vi "Add Field to Image.vi"(9 "Terminal Info":T1, 10 "location":i16=1, 11 "picture":picture) -> (3 "new picture":picture)   [LabVIEW 2015, in "LVJSON.lvlib" / "Set Object Parameters.xnode"]
uses:
  Set Object Parameters.xnode
  offsets.vi
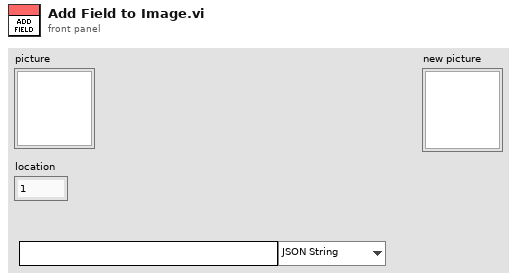
[diagram p1: front panel]
types:
  T1 = cluster{"Parameter Name":string, "JSON Type":enum16{"JSON String", "JSON Numeric", "JSON Boolean", "JSON", "JSON Object", "JSON Array", "String Value", "Numeric Value", "Boolean Value"}}
  T2 = enum16{"User-specified Font", "Application Font", "System Font", "Dialog Font"}
  T3 = cluster{"Font Name:":string, "Size":i16, "Strikeout?":bool, "Italic?":bool, "Underline?":bool, "Outline?":bool, "Shadow?":bool, "Bold?":bool}
  T4 = cluster{"left":i16, "top":i16, "right":i16, "bottom":i16}
  T5 = enum16{"JSON String", "JSON Numeric", "JSON Boolean", "JSON", "JSON Object", "JSON Array", "String Value", "Numeric Value", "Boolean Value"}
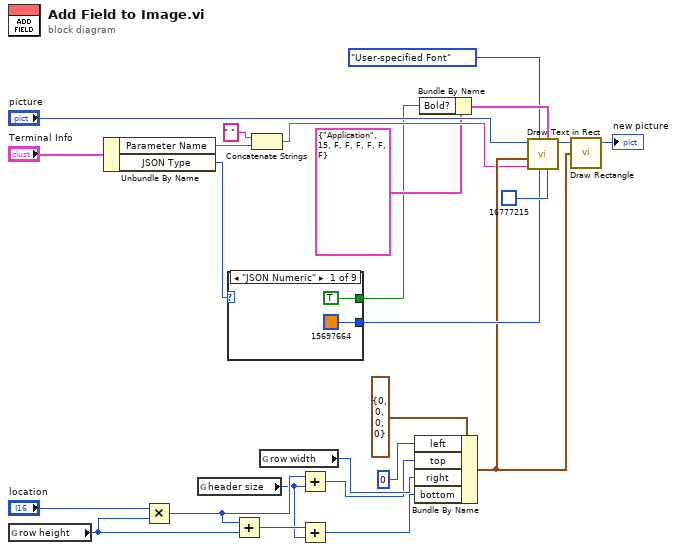
[diagram p0: block diagram]
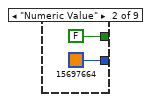
[diagram p2: hidden frame]
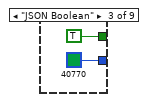
[diagram p3: hidden frame]
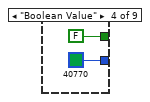
[diagram p4: hidden frame]
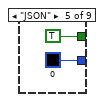
[diagram p5: hidden frame]
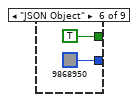
[diagram p6: hidden frame]
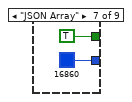
[diagram p7: hidden frame]
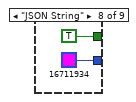
[diagram p8: hidden frame]
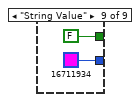
[diagram p9: hidden frame]
diagram:
  n1 = global read "offsets.vi" "row height"() -> (w22:i16)
  n2 = Unbundle By Name("Terminal Info") -> ("Parameter Name"=w7:string, "JSON Type"=w12:T5)
  n3 = Multiply(x="location", y=w22) -> (x*y=w17:i16)
  n4 = global read "offsets.vi" "header size"() -> (w16:i16)
  n5 = case shown="\"JSON Numeric\"" w12 {
    tunnel: [u32 15697664 ("text color(black)") u32 15697664 ("text color(black)") u32 40770 ("text color(black)") u32 40770 ("text color(black)") u32 0 ("text color(black)") u32 9868950 ("text color(black)") u32 16860 ("text color(black)") u32 16711934 ("text color(black)") u32 16711934 ("text color(black)")] -> w10
    tunnel: [TRUE FALSE TRUE FALSE TRUE TRUE TRUE TRUE FALSE] -> w3
    frame "JSON Numeric" {
    }
    frame "Numeric Value" {
    }
    frame "JSON Boolean" {
    }
    frame "Boolean Value" {
    }
    frame "JSON" {
    }
    frame "JSON Object" {
    }
    frame "JSON Array" {
    }
    frame "JSON String" {
    }
    frame "String Value" {
    }
  }
  n6 = Add(x=w17, y=w22) -> (x+y=w19:i16)
  n7 = Concatenate Strings(" " ("string"), w7) -> (w6:string)
  n8 = global read "offsets.vi" "row width"() -> (w21:i16)
  n9 = Add(x=w17, y=w16) -> (x+y=w15:i16)
  n10 = Add(x=w19, y=w16) -> (x+y=w18:i16)
  n11 = Bundle By Name(cluster=T4 {"left"=0, "top"=0, "right"=0, "bottom"=0} ("rect"), "left"=i16 0, "top"=w15, "right"=w21, "bottom"=w18) -> (w9:T4)
  n12 = Bundle By Name(cluster=T3 {"Font Name:"="Application", "Size"=15, "Strikeout?"=FALSE, "Italic?"=FALSE, "Underline?"=FALSE, "Outline?"=FALSE, "Shadow?"=FALSE, "Bold?"=FALSE} ("[user-specified font]"), "Bold?"=w3) -> (w2:T3)
  n13 = call <vilib>:"Draw Text in Rect.vi"("BG color(transparent)"=u32 16777215, "[user-specified font]"=w2, "text color(black)"=w10, "desired font(Application)"=T2."User-specified Font", "text"=w6, "rect"=w9, "picture"="picture") -> ("new picture"=w13:picture)  [unwired: 4 in]
  n14 = call <vilib>:"Draw Rectangle.vi"("picture"=w13, "rect"=w9) -> ("new picture"=→"new picture":picture)  [unwired: 7 in]
